vi "Run Filter Wheel.vi"(8 "error in (no error)":errorcluster, 11 "SPARC4_GEI in":refnum<class "SPARC4_GEI.lvclass">) -> (0 "error out":errorcluster, 3 "SPARC4_GEI out":refnum<class "SPARC4_GEI.lvclass">)   [LabVIEW 2018, in "SPARC4_GEI.lvclass"]
uses:
  SPARC4_GEI.lvclass
  SPARC4_GEI.lvclass/SPARC4_GEI.ctl
  Filter_Wheel/Filter_Wheel.lvclass
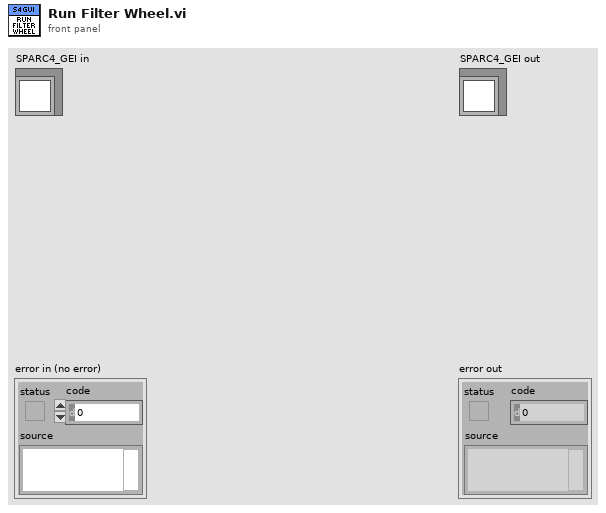
[diagram p1: front panel]
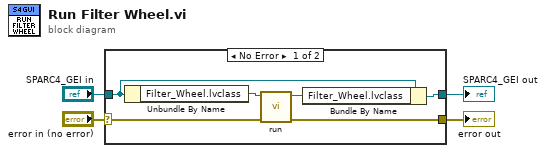
[diagram p0: block diagram]
diagram:
  n1 = case shown="No Error" "error in (no error)" {
    selector: "error in (no error)" -> [w9 w12]
    tunnel: [w5 w12] -> w3
    tunnel: [w7 w11] -> w1
    tunnel: "SPARC4_GEI in" -> [w8 w11]
    frame No Error {
      n2 = Unbundle By Name(w8) -> ("Filter_Wheel.lvclass"=w10:refnum<class "Filter_Wheel.lvclass">)
      n3 = call "run.vi"("error in (no error)"=w9, "Filter_Wheel in"=w10) -> ("error out"=w5:errorcluster, "Filter_Wheel out"=w6:refnum<class "Filter_Wheel.lvclass">)  [unwired: 8 in]
      n4 = Bundle By Name(cluster=w8, "Filter_Wheel.lvclass"=w6) -> (w7:refnum<class "SPARC4_GEI.lvclass">)
    }
    frame Error {
    }
  }
  "error out" <- w3
  "SPARC4_GEI out" <- w1
